vi "start listening.vi"(8 "error in":errorcluster, 11 "Queue server in":refnum<class "Queue server.lvclass">) -> (0 "error out":errorcluster, 3 "Queue server out":refnum<class "Queue server.lvclass">)   [LabVIEW 2015, in "Queue server.lvclass"]
uses:
  Queue server.lvclass
  message/communicator message.lvclass
  server/connection server.lvclass/connection server.ctl
  Queue server.lvclass/Queue server.ctl
  server/connection server.lvclass
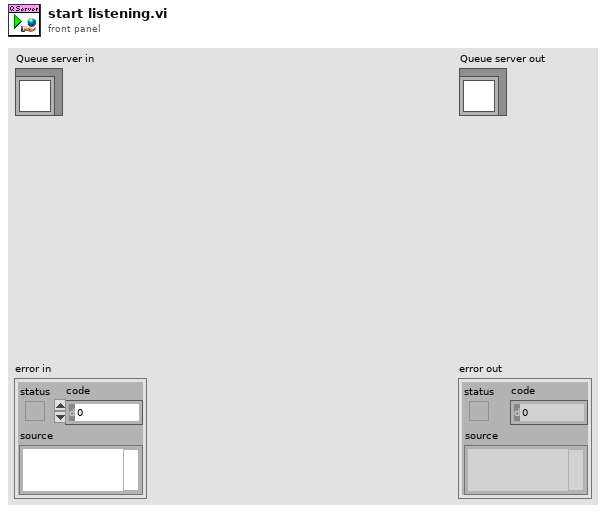
[diagram p1: front panel]
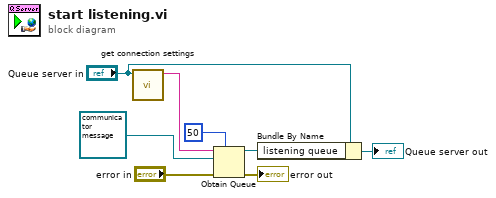
[diagram p0: block diagram]
diagram:
  n1 = call "get connection settings.vi"("connection server in"="Queue server in") -> ("connection string"=w1:string)  [unwired: 9 in, 1 out]
  n2 = Obtain Queue(max queue size (-1, unlimited)=50, name (unnamed)=w1, element data type=refnum<class "communicator message.lvclass"> refnum ("communicator message.lvclass"), error in (no error)="error in") -> (queue out=w3:refnum<queue>, error out=→"error out":errorcluster)  [unwired: 1 in, 1 out]
  n3 = Bundle By Name(cluster="Queue server in", "listening queue"=w3) -> (→"Queue server out":refnum<class "Queue server.lvclass">)
